vi "Osciloscopio.vi"() -> ()   [LabVIEW 2020]
panel:
  in  "stop (F)":bool
  in  "Frequency":dbl=10.1
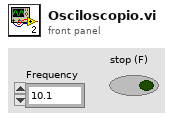
[diagram p1: front panel]
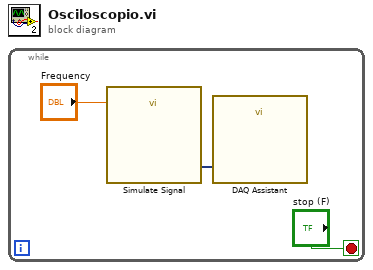
[diagram p0: block diagram]
diagram:
  n1 = while {
    stop <- "stop (F)" stop-if-true
    n2 = call "Simulate Signal"("Frequency"="Frequency") -> ("Sine"=w3:dynamicdata)  [unwired: 13 in, 1 out]
    n3 = call "DAQ Assistant"("data"=w3) -> ()  [unwired: 17 in, 2 out]
  }
